vi "DiscArchiver.get alarm level.vi"(0 "i ref in":refnum<vi>, 5 "error in (no error)":errorcluster) -> (14 "i ref out":refnum<vi>, 16 "alarm level":dbl format="%.2f", 19 "error out":errorcluster)   [LabVIEW 2014, in "DiscArchiver.lvlib"]
doc: "Gets the alarm level for the \"free disc\" fraction. Example: An alarm level of 0.1 corresponds to 10% of the available disc size."
uses:
  DiscArchiver.lvlib
  CSCore/BaseProcess/BaseProcess.lvlib
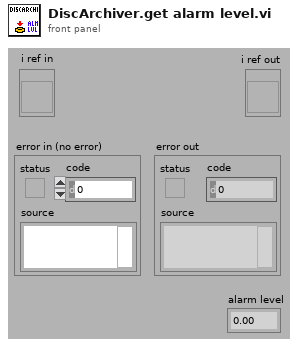
[diagram p1: front panel]
types:
  T1 = typedef "BaseProcess.lvlib/BaseProcess.i attribute.ctl" = cluster{"EventStatus":string, "EventError":i32, "PresetEvtWatchD":i32, "PresetPdcWatchD":i32, "EventTimeout":i32, "PeriodicInterval":i32, "Interface":string[], "Address":string[], "Special":string[], "PeriodicError":i32, "PeriodicStatus":string, "SuperProc":string, "Descriptors":T2[], "CaseRef":refnum<vi>, "PdcRef":refnum<vi>, "Thread Ref":refnum<vi>, "eventErrorID":i32, "eventStatusID":i32, "periodicErrorID":i32, "periodicStatusID":i32, "pdcCtrID":i32}
  T2 = typedef "BaseProcess.lvlib/BaseProcess.descriptor definition.ctl" = cluster{"selector":string, "descriptor":T3}
  T3 = typedef "BaseProcess.lvlib/BaseProcess.descriptor string definition.ctl" = string
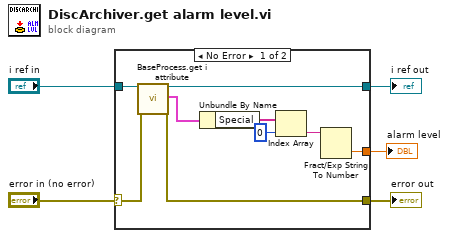
[diagram p0: block diagram]
diagram:
  n1 = case shown="No Error" "error in (no error)" {
    selector: "error in (no error)" -> [w6 w15]
    tunnel: "i ref in" -> [w14 w16]
    tunnel: [w12 w15] -> w4
    tunnel: [w11 w16] -> w3
    tunnel: [w7 _] -> w2
    frame No Error {
      n2 = call "BaseProcess.get i attribute.vi"("i ref in"=w14, "error in (no error)"=w6) -> ("i ref out"=w11:refnum<vi>, "i attribute"=w13:T1, "error out"=w12:errorcluster)  [unwired: 15 in]
      n3 = Unbundle By Name(w13) -> ("Special"=w10:string[])
      n4 = Index Array(array=w10, index=0) -> (element=w8:string)
      n5 = Fract/Exp String To Number(string=w8) -> (number=w7:dbl)  [unwired: 3 in, 1 out]
    }
    frame Error {
    }
  }
  "error out" <- w4
  "i ref out" <- w3
  "alarm level" <- w2
